vi "Acquire Semaphore.vi"(8 "error in (no error)":errorcluster, 10 "VI Refnum in":refnum<vi>, 11 "Slave Test Runner in":refnum<class "Slave Test Runner.lvclass">) -> (0 "error out":errorcluster, 2 "VI Refnum out":refnum<vi>, 3 "Slave Test Runner out":refnum<class "Slave Test Runner.lvclass">)   [LabVIEW 2020, in "Slave Test Runner.lvclass"]
doc: "Wait for the method to become available for execution when running tests in parallell."
uses:
  Slave Test Runner.lvclass
  Slave Test Runner.lvclass/Slave Test Runner.ctl
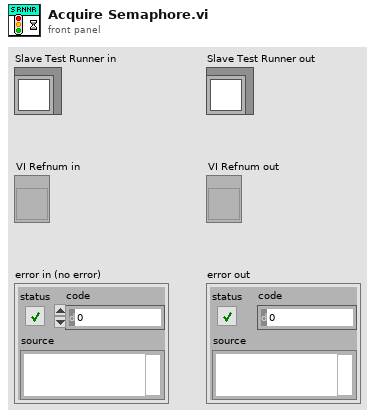
[diagram p1: front panel]
types:
  T1 = typedef "Semaphore RefNum" = refnum<k1>
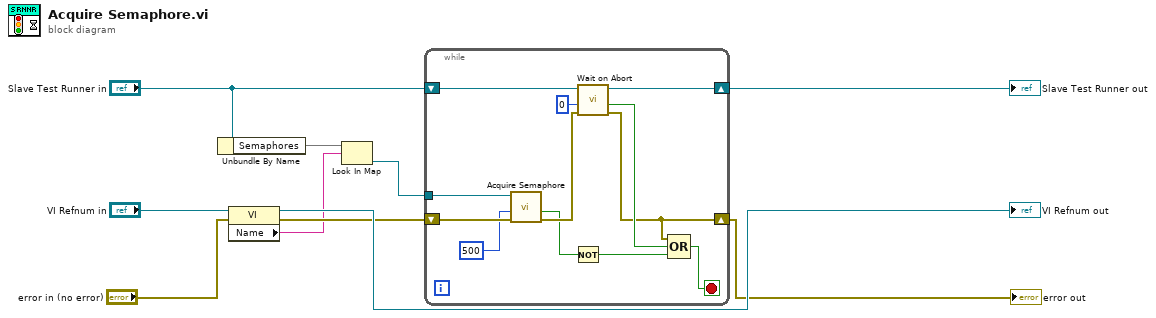
[diagram p0: block diagram]
diagram:
  n1 = Unbundle By Name("Slave Test Runner in") -> ("Semaphores"=w2:map{string, T1})
  n2 = property on="Property Node" class="VI"(reference="VI Refnum in", error in="error in (no error)") -> (reference out=→"VI Refnum out":refnum<vi>, error out=w4:errorcluster, "Name"=w1:string)
  n3 = Look In Map(map=w2, key=w1) -> (value=w3:T1)  [unwired: 1 in, 1 out]
  n4 = while {
    shift-right: [w22] -> w10
    shift-left: "Slave Test Runner in" -> [w21]
    shift-right: [w11] -> w5
    shift-left: w4 -> [w20]
    tunnel: w3 -> [w12]
    stop <- w13 stop-if-true
    n5 = call <vilib>:"Acquire Semaphore.vi"("error in (no error)"=w20, "ms timeout (-1)"=500 ("timeout in ms (0)"), "semaphore"=w12) -> ("error out"=w17:errorcluster, "timed out"=w16:bool)  [unwired: 2 in, 1 out]
    n6 = Not(x=w16) -> (.not. x?=w15:bool)
    n7 = call "Wait on Abort.vi"("error in (no error)"=w17, "timeout in ms (0)"=0, "Slave Test Runner In"=w21) -> ("error out"=w11:errorcluster, "Aborted?"=w14:bool, "Slave Test Runner Out"=w22:refnum<class "Slave Test Runner.lvclass">)  [unwired: 6 in]
    n8 = Compound Arithmetic op=OR(w11, w14, w15) -> (w13:bool)
  }
  "Slave Test Runner out" <- w10
  "error out" <- w5
